vi "open fpga cal refs.vi"(8 "Error In":errorcluster, 11 "Top level fpga ref":refnum<k20>) -> (0 "Error out":errorcluster, 1 "Cal offset refs":refnum<k20>[](array[refnum]), 2 "Cal input refs":refnum<k20>[](array[refnum]), 3 "Top level fpga ref":refnum<k20>)   [LabVIEW 2014]
uses:
  <vilib>/NI/LVFPGA Adv Session Resources/OpenByNameSubVI.vi
  Shared/Constants.vi
  <vilib>/rvi/interface/common/dynamic/niFpgaEscapeDelimiterAndNull.vi
  <vilib>/Utility/error.llb/Error Cluster From Error Code.vi
  <vilib>/NI/LVFPGA Adv Session Resources/OpenByName.xnode
  <vilib>/NI/LVFPGA Adv Session Resources/LVFPGAAdvSessionResources.lvlib
  Shared/UEGO Sim Shared.lvlib
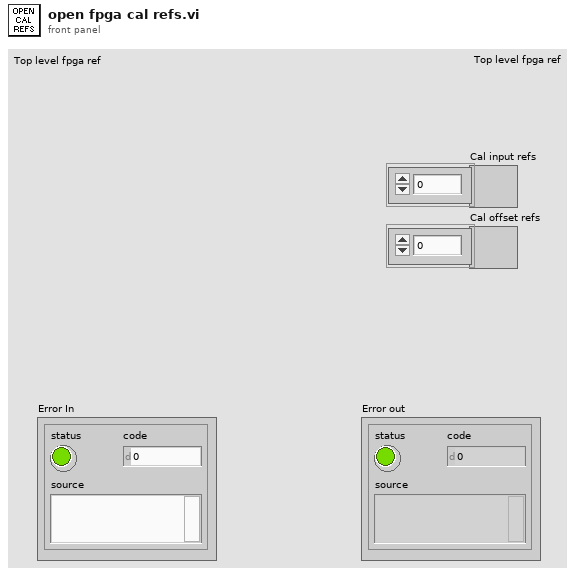
[diagram p1: front panel]
types:
  T1 = cluster{"Name":string, "Depth":u32, "Write? (Deprecated:Use Implementation)":bool, "Physical Channel":u32, "Base Address":u32, "Data Width":u32, "Data Type":enum32{"Boolean", "I8", "I16", "I32", "I64", "U8", "U16", "U32", "U64", "FXP", "CustomControl", "SGL"}, "FXP Properties":variant, "Write Window Address":u32, "Implementation":enum16{"niFpgaTargetToHost", "niFpgaHostToTarget", "niFpgaPeerToPeerWriter", "niFpgaPeerToPeerReader", "niCoreTargetToHost", "niCoreHostToTarget"}, "Control Set":u32}[]
  T2 = cluster{"Name":string, "type":variant, "indicator?":bool}[]
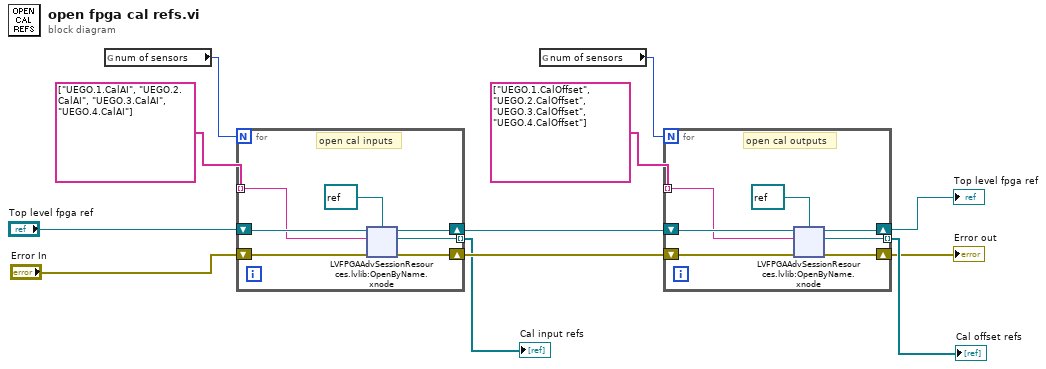
[diagram p0: block diagram]
diagram:
  n1 = global read "Constants.vi" "num of sensors"() -> (w11:i32)
  n2 = for {
    N: w11 -> [_]
    tunnel: string[] ["UEGO.1.CalAI", "UEGO.2.CalAI", "UEGO.3.CalAI", "UEGO.4.CalAI"] -> [w17] mode=indexing
    tunnel: [w15] -> w5 mode=indexing
    shift-right: [w14] -> w6
    shift-left: "Error In" -> [w18]
    shift-right: [w13] -> w7
    shift-left: "Top level fpga ref" -> [w19]
    # "open cal inputs"
    n3 = xnode "LVFPGAAdvSessionResources.lvlib:OpenByName.xnode"("FPGA VI Reference in"=w19, "Resource name in"=w17, "Single resource reference type in"=refnum<k20> refnum, "Error in"=w18) -> ("Single resource reference out"=w15:refnum<k20>, "Error out"=w14:errorcluster, "FPGA VI Reference out"=w13:refnum<k20>)
  }
  "Cal input refs" <- w5
  n4 = global read "Constants.vi" "num of sensors"() -> (w10:i32)
  n5 = for {
    N: w10 -> [_]
    tunnel: string[] ["UEGO.1.CalOffset", "UEGO.2.CalOffset", "UEGO.3.CalOffset", "UEGO.4.CalOffset"] -> [w37] mode=indexing
    tunnel: [w35] -> w4 mode=indexing
    shift-right: [w34] -> w1
    shift-left: w6 -> [w38]
    shift-right: [w33] -> w2
    shift-left: w7 -> [w39]
    # "open cal outputs"
    n6 = xnode "LVFPGAAdvSessionResources.lvlib:OpenByName.xnode"("FPGA VI Reference in"=w39, "Resource name in"=w37, "Single resource reference type in"=refnum<k20> refnum, "Error in"=w38) -> ("Single resource reference out"=w35:refnum<k20>, "Error out"=w34:errorcluster, "FPGA VI Reference out"=w33:refnum<k20>)
  }
  "Cal offset refs" <- w4
  "Top level fpga ref" <- w2
  "Error out" <- w1
